vi "imageResize.vi"(2 "colScale":i32, 3 "rowScale":i32, 4 "image":u8[][](array[numeric])) -> (0 "resized image":u8[][](array[numeric]))   [LabVIEW 2016]
uses:
  <vilib>/Analysis/7linalg.llb/Real Kronecker Product.vi
  <vilib>/Analysis/NI_AALPro.lvlib
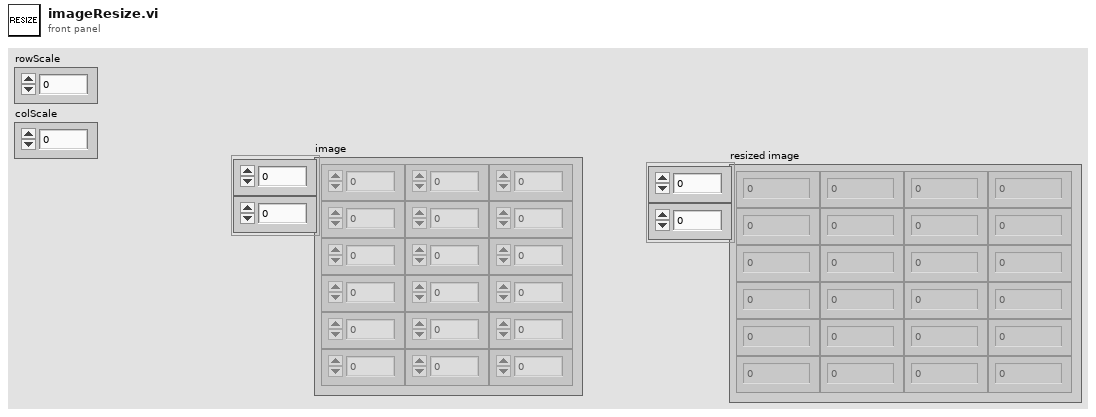
[diagram p1: front panel]
types:
  T1 = typedef "NI_Matrix.lvlib/RealMatrix.ctl" = dbl[][]
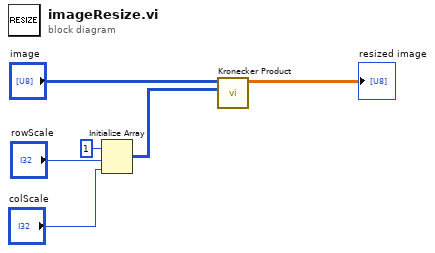
[diagram p0: block diagram]
diagram:
  n1 = Initialize Array(u8 1 ("element"), "rowScale", "colScale") -> (w3:u8[][])
  n2 = call-poly <vilib>:"Kronecker Product.vi"("B"=w3, "A"="image") -> ("Kronecker Product"=→"resized image":T1)  [unwired: 8 in, 1 out]
